vi "Select System By Chnl.vi"(8 "error in (no error)":errorcluster, 10 "ChnlName":string, 11 "SystemsIn":refnum<class "BME_DG_System.lvclass">[](array[class])) -> (0 "error out":errorcluster, 1 "BME_DG_Chnl":refnum<class "BME_DG_Chnl.lvclass">, 2 "BME_DG_System out":refnum<class "BME_DG_System.lvclass">, 3 "SystemsOut":refnum<class "BME_DG_System.lvclass">[](array[class]), 4 "Owner DG":refnum<class "BME_DG_Base.lvclass">)   [LabVIEW 2009, in "POLARIS BME DG.lvlib" / "BME_DG_System.lvclass"]
uses:
  BME_DG_System.lvclass
  BME_DG_Chnl/BME_DG_Chnl.lvclass
  BME_DG_Base/BME_DG_Base.lvclass
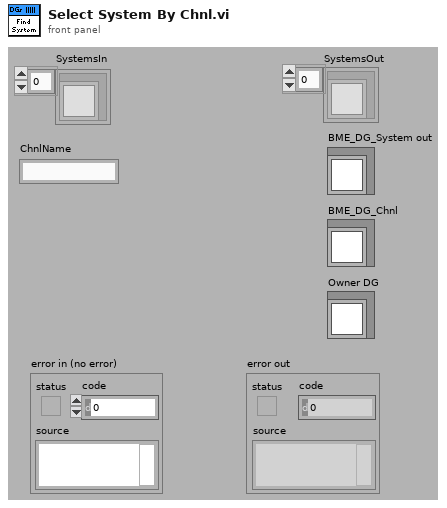
[diagram p1: front panel]
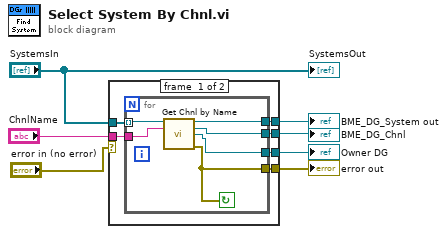
[diagram p0: block diagram]
diagram:
  n1 = case shown="No Error" "error in (no error)" {
    selector: "error in (no error)" -> [_ w20]
    tunnel: "SystemsIn" -> [w13 _]
    tunnel: "ChnlName" -> [w12 _]
    tunnel: [w11 _] -> w5
    tunnel: [w10 w20] -> w4
    tunnel: [w9 _] -> w2
    tunnel: [w8 _] -> w1
    frame #0 {
      n2 = for {
        tunnel: w13 -> [w19] mode=indexing
        tunnel: w12 -> [w18]
        tunnel: [w17] -> w11
        tunnel: [w16] -> w10
        tunnel: [w15] -> w9
        tunnel: [w14] -> w8
        stop <- w16 continue-if-true
        n3 = call "Get Chnl by Name.vi"("BME_DG_System in"=w19, "Chnl Name"=w18) -> ("BME_DG_System out"=w17:refnum<class "BME_DG_System.lvclass">, "BME_DG_Chnl"=w15:refnum<class "BME_DG_Chnl.lvclass">, "Owner DG"=w14:refnum<class "BME_DG_Base.lvclass">, "error out"=w16:errorcluster)  [unwired: 8 in, 2 out]
      }
    }
    frame #1 {
    }
  }
  "error out" <- w4
  "BME_DG_System out" <- w5
  "BME_DG_Chnl" <- w2
  "Owner DG" <- w1
  "SystemsOut" <- "SystemsIn"
